vi "sub_createAOwave.vi"(11 "AO signal":T1={"offset"=1.0, "signal type"=enum."Square Wave", "frequency"=10.0, "amplitude"=1.0, " duty"=50.0} {"amplitude" format="%0.2p"; "frequency" format="%.0p"; "offset" format="%0.2p"}) -> (3 "AO wave":waveform(dbl)(graph)={"t0"=timestamp(0 s since 1904-01-01), "dt"=0.001, "Y"=array[1000 elements]})   [LabVIEW 2019]
uses:
  <vilib>/measure/NI_MABase.lvlib
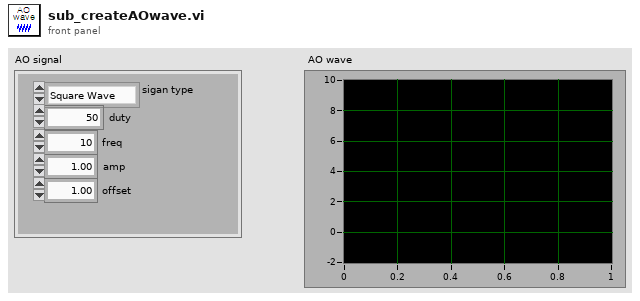
[diagram p1: front panel]
types:
  T1 = cluster{"offset":dbl, "signal type":enum16{"Sine Wave", "Triangle Wave", "Square Wave", "Sawtooth Wave"}, "frequency":dbl, "amplitude":dbl, " duty":dbl}
  T2 = enum16{"Sine Wave", "Triangle Wave", "Square Wave", "Sawtooth Wave"}
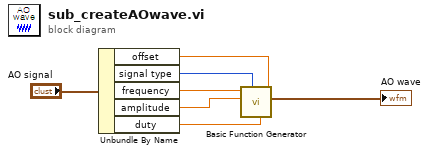
[diagram p0: block diagram]
diagram:
  n1 = Unbundle By Name("AO signal") -> ("offset"=w5:dbl, "signal type"=w6:T2, "frequency"=w4:dbl, "amplitude"=w3:dbl, "duty"=w2:dbl)
  n2 = call <vilib>:"Basic Function Generator.vi"("offset"=w5, "square wave duty cycle (%)"=w2, "signal type"=w6, "amplitude"=w3, "frequency"=w4) -> ("signal out"=→"AO wave":waveform(dbl))  [unwired: 4 in, 2 out]
